vi "MainPresentor.vi"() -> ()   [LabVIEW 2010]
uses:
  <vilib>/Utility/miscctls.llb/LV3DPointTypeDef.ctl
  LVPresent_Globals.vi
panel:
  out "queue":string
  out "ScanCode":i16
  out "3D Picture":refnum<vi>(3d-picture)
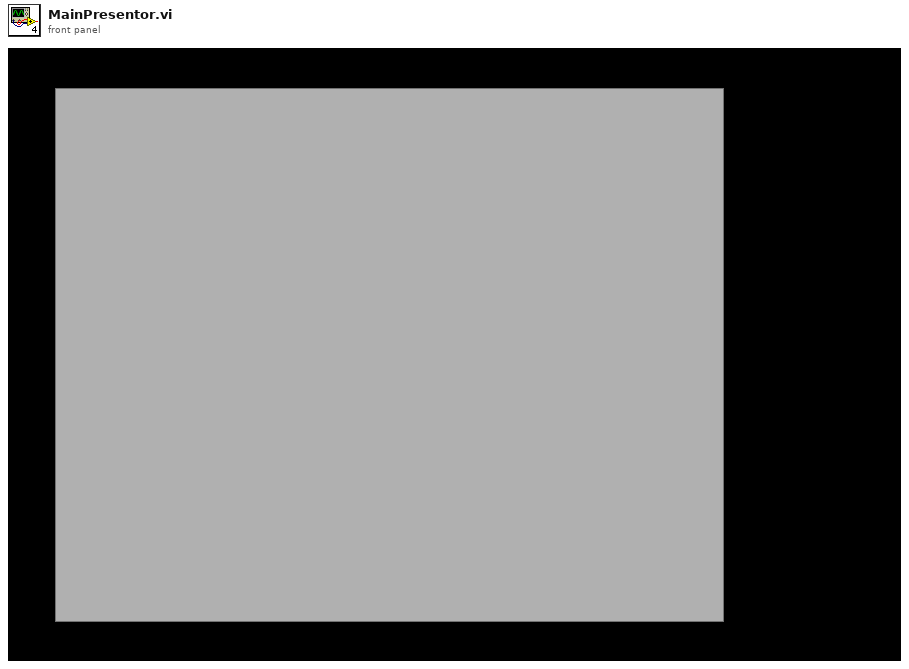
[diagram p1: front panel]
types:
  T1 = typedef "LV3DPointTypeDef.ctl" = cluster{"X":sgl, "Y":sgl, "Z":sgl}
  T2 = typedef "LVBoundsTypeDef.ctl" = cluster{"Width":u32, "Height":u32}
  T3 = typedef "LVRectTypeDef.ctl" = cluster{"left":i16, "top":i16, "right":i16, "bottom":i16}
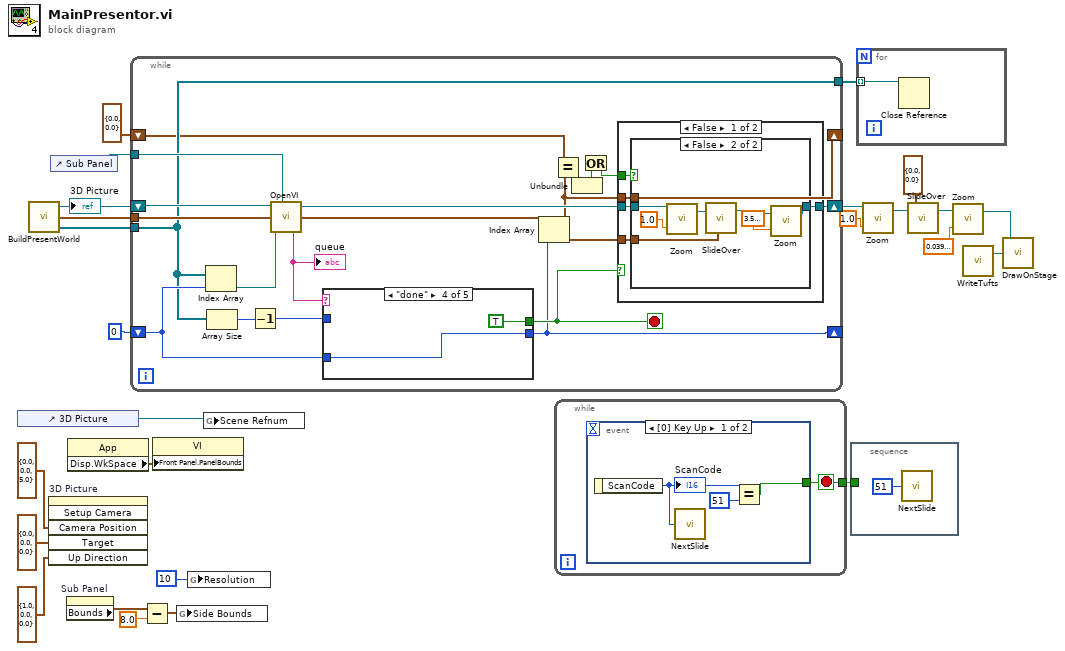
[diagram p0: block diagram]
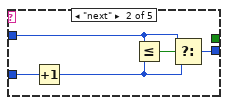
[diagram p3: hidden frame]
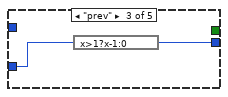
[diagram p4: hidden frame]
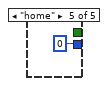
[diagram p5: hidden frame]
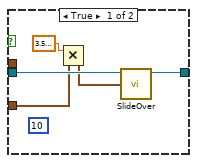
[diagram p6: hidden frame]
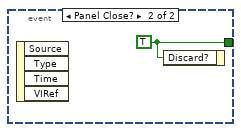
[diagram p8: hidden frame]
diagram:
  n1 = control-ref of="3D Picture"() -> (w2:refnum<vi>)
  n2 = call "BuildPresentWorld.vi"() -> ("Array"=w22:refnum<vi>[], "positions"=w14:cluster{"X":sgl, "Y":sgl}[], "Scene.Object Out"=w19:refnum<vi>)  [unwired: 2 in]
  "3D Picture" <- w19
  n3 = invoke on="3D Picture" class="SceneGraphDisp (strict)" method="Setup Camera"("Camera Position"=T1 {"X"=0.0, "Y"=0.0, "Z"=5.0}, "Target"=T1 {"X"=0.0, "Y"=0.0, "Z"=0.0}, "Up Direction"=T1 {"X"=1.0, "Y"=0.0, "Z"=0.0}) -> ()  [unwired: 3 in, 6 out]
  n4 = control-ref of="Sub Panel"() -> (w18:refnum<vi>)
  n5 = property on="Sub Panel" class="SubPnl"() -> ("Bounds"=w4:T2)  [unwired: 2 in, 2 out]
  n6 = property class="App"() -> ("Disp.WkSpace"=w6:T3)  [unwired: 2 in, 2 out]
  n7 = while {
    shift-right: [w44] -> w17
    shift-left: w19 -> [w43]
    tunnel: w22 -> [w32]
    tunnel: w18 -> [w42]
    shift-right: [w33] -> _
    shift-left: 0 ("Resolution") -> [w34]
    tunnel: w14 -> [w35]
    tunnel: [w32] -> w12
    shift-right: [w30] -> _
    shift-left: cluster{"X":sgl, "Y":sgl} {"X"=0.0, "Y"=0.0} -> [w31]
    stop <- w36 stop-if-true
    n8 = Index Array(array=w32, index=w34) -> (element=w39:refnum<vi>)
    n9 = Array Size(array=w32) -> (size(s)=w38:i32)
    n10 = Decrement(x=w38) -> (x-1=w37:i32)
    n11 = call "OpenVI.vi"("Scene.Object in"=w43, "reference"=w42, "vi reference"=w39) -> ("Scene.Object Out"=w41:refnum<vi>, "queue"=w40:string)  [unwired: 3 in]
    "queue" <- w40
    n12 = case shown="\"done\"" w40 {
      tunnel: [w45 w47 w51 w53 0 ("Resolution")] -> w33
      tunnel: w34 -> [w45 w50 w52 w53 _]
      tunnel: [_ _ _ TRUE _] -> w36
      tunnel: w37 -> [_ w48 _ _ _]
      frame Default {
      }
      frame "next" {
        n13 = Increment(x=w50) -> (x+1=w46:i32)
        n14 = Less Or Equal?(x=w48, y=w46) -> (x <= y?=w49:bool)
        n15 = Select(t=w48, s=w49, f=w46) -> (s? t:f=w47:i32)
      }
      frame "prev" {
        n16 = expression code="x>1?x-1:0"(w52) -> (w51:i32)
      }
      frame "done" {
      }
      frame "home" {
      }
    }
    n17 = Index Array(array=w35, index=w33) -> (element=w30:cluster{"X":sgl, "Y":sgl})
    n18 = Equal?(x=w31, y=w30) -> (x = y?=w29:cluster{"X":bool, "Y":bool})
    n19 = Unbundle(w29) -> ("X"=w28:bool, "Y"=w27:bool)
    n20 = Or(x=w28, y=w27) -> (x .or. y?=w26:bool)
    n21 = case shown="False" w36 {
      tunnel: [w58 w73] -> w44
      tunnel: w41 -> [w59 w73]
      tunnel: w30 -> [w60 _]
      tunnel: w26 -> [w57 _]
      tunnel: w30 -> [w56 _]
      frame False {
        n22 = case shown="False" w57 {
          tunnel: w60 -> [w62 w72]
          tunnel: w59 -> [w64 w70]
          tunnel: [w65 w67] -> w58
          tunnel: w56 -> [_ _]
          frame True {
            (unwired) 10 ("Resolution")
            n23 = Multiply(x=sgl 3.6 ("Final Zoom"), y=w62) -> (x*y=w61:cluster{"X":sgl, "Y":sgl})
            n24 = call "SlideOver.vi"("Scene.Object IN"=w64, "Position"=w61) -> ("Scene.Object Out"=w65:refnum<vi>)  [unwired: 4 in]
          }
          frame False {
            n25 = call "Zoom.vi"("Final Zoom"=sgl 1.0, "Scene.Object IN"=w70) -> ("Scene.Object Out"=w69:refnum<vi>)  [unwired: 1 in]
            n26 = call "SlideOver.vi"("Position"=w72, "Scene.Object IN"=w69) -> ("Scene.Object Out"=w68:refnum<vi>)  [unwired: 1 in]
            n27 = call "Zoom.vi"("Final Zoom"=sgl 3.6, "Scene.Object IN"=w68) -> ("Scene.Object Out"=w67:refnum<vi>)  [unwired: 1 in]
          }
        }
      }
      frame True {
      }
    }
  }
  n28 = Subtract(x=w4, y=8.0) -> (x-y=w3:cluster{"Width":dbl, "Height":dbl})
  n29 = property class="VI"("Front Panel.PanelBounds"=w6) -> ()  [unwired: 2 in, 2 out]
  n30 = global write "LVPresent_Globals.vi" "Side Bounds"(w3) -> ()
  n31 = global write "LVPresent_Globals.vi" "Resolution"(10 ("Resolution")) -> ()
  n32 = global write "LVPresent_Globals.vi" "Scene Refnum"(w2) -> ()
  n33 = while {
    tunnel: [w74] -> w20
    stop <- w74 stop-if-true
    n34 = event shown="[0] Key Up" {
      selector: _ -> [_ _]
      dyn-events: _ -> [_ _]
      timeout: _ -> [_ _]
      tunnel: [w76 w78] -> w74
      event Key Up {
        n35 = event-data() -> ("ScanCode"=w77:i16)  [unwired: 1 in]
        "ScanCode" <- w77
        n36 = call "NextSlide.vi"("ScanCode"=w77) -> ()
        n37 = Equal?(x=w77, y=i16 51 ("ScanCode")) -> (x = y?=w76:bool)
      }
      event Panel Close? {
        w78 = TRUE
        n38 = event-data() -> ()  [unwired: 1 in, 4 out]
        n39 = event-data("Discard?"=w78) -> ()  [unwired: 1 in, 1 out]
      }
    }
  }
  n40 = stacked-sequence {
    tunnel: w20 -> [_]
    frame #0 {
      n41 = call "NextSlide.vi"("ScanCode"=i16 51) -> ()
    }
  }
  n42 = for {
    tunnel: w12 -> [w80] mode=indexing
    n43 = Close Reference(reference=w80) -> ()  [unwired: 1 in, 1 out]
  }
  n44 = call "Zoom.vi"("Final Zoom"=sgl 1.0, "Scene.Object IN"=w17) -> ("Scene.Object Out"=w16:refnum<vi>)  [unwired: 1 in]
  n45 = call "SlideOver.vi"("Position"=cluster{"X":sgl, "Y":sgl} {"X"=0.0, "Y"=0.0}, "Scene.Object IN"=w16) -> ("Scene.Object Out"=w10:refnum<vi>)  [unwired: 1 in]
  n46 = call "Zoom.vi"("Final Zoom"=sgl 0.04, "Scene.Object IN"=w10) -> ("Scene.Object Out"=w7:refnum<vi>)  [unwired: 1 in]
  n47 = call "WriteTufts.vi"() -> ("Scene.Object Out"=w8:refnum<vi>)  [unwired: 1 in]
  n48 = call <userlib>:"DrawOnStage.vi"("object in"=w8, "Stage in"=w7) -> ()  [unwired: 1 in, 3 out]
